vi "ui_DataLog Query Meta.vi"(7 "base tag":string) -> (3 "initial value out":dbl format="%.2f", 4 "OKed?":bool, 8 "meta out":T1)   [LabVIEW 2012]
doc: "This dialog queries meta tag type and initial value."
uses:
  typedefs/et_DataLog Meta Tag Specifier.ctl
  typedefs/t_DataLog Query Meta States.ctl
panel:
  in  "initial value":dbl format="%.4e"
  in  "meta specifier":T1=enum."not a meta"
  in  "cancel":bool
  in  "OK":bool
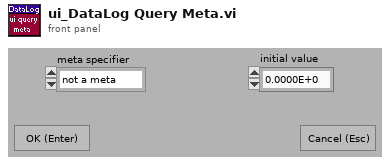
[diagram p1: front panel]
types:
  T1 = typedef "et_DataLog Meta Tag Specifier.ctl" = enum32{"warn_lo", "warn_hi", "A_lo", "A_hi", "B_lo", "B_hi", "C_lo", "C_hi", "D_lo", "D_hi", "E_lo", "E_hi", "F_lo", "F_hi", "G_lo", "G_hi", "H_lo", "H_hi", "I_lo", "I_hi", "J_lo", "J_hi", "K_lo", "K_hi", "L_lo", "L_hi", "M_lo", "M_hi", "N_lo", "N_hi", "min", "max", "not a meta"}
  T2 = typedef "t_DataLog Query Meta States.ctl" = enum16{"empty queue", "initialize", "stop"}
  T3 = typedef "eventvkey.ctl" = enum16{"ASCII", "Enter", "Return", "Shift", "Ctrl", "Alt", "Cmd", "Opt", "Caps", "NumLock", "Clear", "Break", "Up", "Down", "Left", "Right", "Insert", "Delete", "Home", "End", "PageUp", "PageDown", "Escape", "Help", "Pause", "ScrollLock", "F1", "F2", "F3", "F4", "F5", "F6", "F7", "F8", "F9", "F10", "F11", "F12", "F13", "F14", "F15", "F16", "F17", "F18", "F19", "F20", "F21", "F22", "F23", "F24", "Play", "VolumeUp", "VolumeDown", "Mute", "Two Byte Char"}
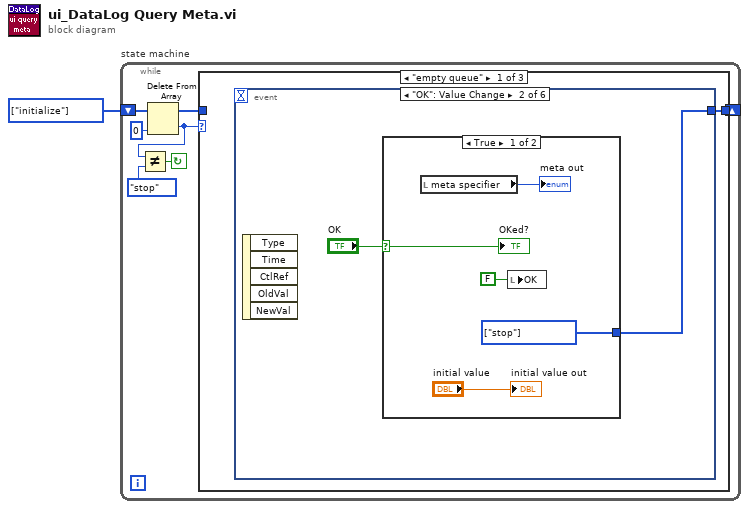
[diagram p0: block diagram]
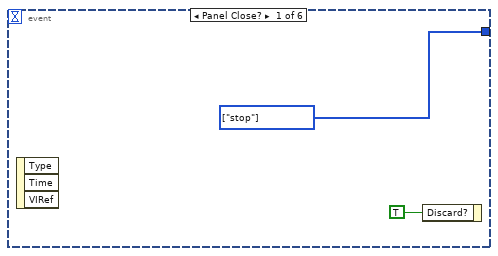
[diagram p2: hidden frame]
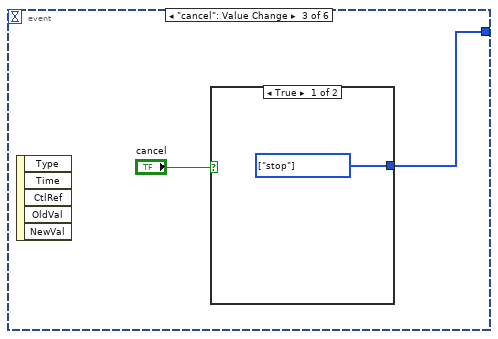
[diagram p4: hidden frame]
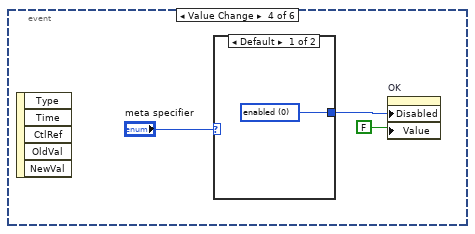
[diagram p6: hidden frame]
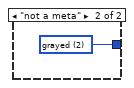
[diagram p7: hidden frame]
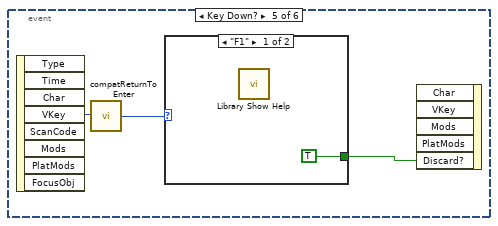
[diagram p8: hidden frame]
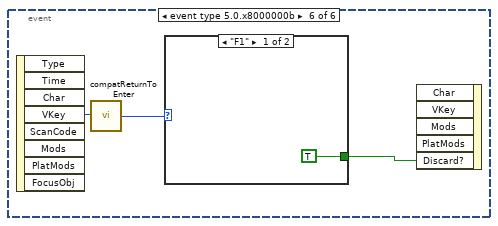
[diagram p10: hidden frame]
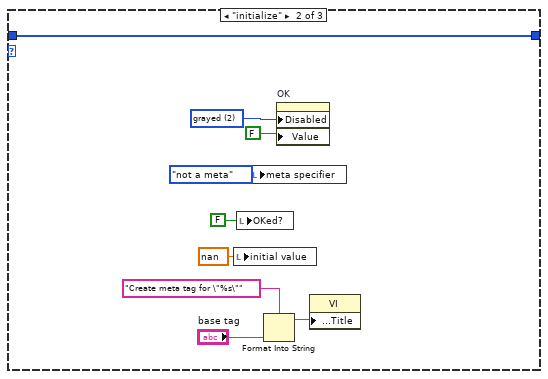
[diagram p12: hidden frame]
diagram:
  w1 = T2[] [enum."initialize"] items=["empty queue", "initialize", "stop"] ("Array Constant")
  n1 = while "state machine" {
    shift-left: w1 -> [w5]
    shift-right: [w8] -> _
    stop <- w7 continue-if-true
    n2 = Delete From Array(array=w5, index=0) -> (deleted portion=w3:T2, array with subset deleted=w4:T2[])  [unwired: 1 in]
    n3 = Not Equal?(x=w3, y=t_DataLog_Query_Meta_States."stop" ("states")) -> (x != y?=w7:bool)
    n4 = case "Case" shown="\"empty queue\"" w3 {
      tunnel: [w9 w43 w44] -> w8
      tunnel: w4 -> [_ w43 w44]
      frame "empty queue" {
        n5 = event shown="[1] \"OK\": Value Change" {
          selector: _ -> [_ _ _ _ _ _]
          dyn-events: _ -> [_ _ _ _ _ _]
          timeout: _ -> [_ _ _ _ _ _]
          tunnel: [w11 w13 w20 _ _ _] -> w9
          event Panel Close? {
            w11 = T2[] [enum."stop"] items=["empty queue", "initialize", "stop"] ("Array Constant")
            n6 = event-data() -> ()  [unwired: 1 in, 3 out]
            n7 = event-data("Discard?"=TRUE) -> ()  [unwired: 1 in, 1 out]
          }
          event "OK": Value Change {
            n8 = event-data() -> ()  [unwired: 1 in, 5 out]
            n9 = case shown="True" "OK" {
              selector: "OK" -> [w17 _]
              tunnel: [w18 _] -> w13
              frame True {
                w18 = T2[] [enum."stop"] items=["empty queue", "initialize", "stop"] ("Array Constant")
                n10 = local read "meta specifier"() -> (→"meta out":T1)
                n11 = local write "OK"(FALSE ("OK")) -> ()
                "OKed?" <- w17
                "initial value out" <- "initial value"
              }
              frame False {
              }
            }
          }
          event "cancel": Value Change {
            n12 = event-data() -> ()  [unwired: 1 in, 5 out]
            n13 = case shown="True" "cancel" {
              tunnel: [w21 _] -> w20
              frame True {
                w21 = T2[] [enum."stop"] items=["empty queue", "initialize", "stop"] ("Array Constant")
              }
              frame False {
              }
            }
          }
          event Value Change {
            n14 = event-data() -> ()  [unwired: 1 in, 5 out]
            n15 = case shown="Default" "meta specifier" {
              tunnel: [w25 w26] -> w22
              frame Default {
                w25 = u8 0 items=["enabled", "disabled", "grayed"] ("disabled state")
              }
              frame "not a meta" {
                w26 = u8 2 items=["enabled", "disabled", "grayed"] ("disabled state")
              }
            }
            n16 = property on="OK" class="Bool (strict)"("Disabled"=w22, "Value"=FALSE ("OK")) -> ()  [unwired: 2 in, 2 out]
          }
          event Key Down? {
            n17 = event-data() -> ("VKey"=w27:T3)  [unwired: 1 in, 7 out]
            n18 = call <vilib>:"compatReturnToEnter.vi"("VKey"=w27) -> ("VKey"=w29:T3)
            n19 = case shown="\"F1\"" w29 {
              tunnel: [TRUE ("Discard?") _] -> w28
              frame "F1" {
                n20 = call "Library Show Help.vi"() -> ()  [unwired: 1 in]
              }
              frame Default {
              }
            }
            n21 = event-data("Discard?"=w28) -> ()  [unwired: 5 in, 1 out]
          }
          event event type 5.0.x8000000b {
            n22 = event-data() -> ("VKey"=w31:T3)  [unwired: 1 in, 7 out]
            n23 = call <vilib>:"compatReturnToEnter.vi"("VKey"=w31) -> ("VKey"=w33:T3)
            n24 = case shown="\"F1\"" w33 {
              tunnel: [TRUE ("Discard?") _] -> w32
              frame "F1" {
              }
              frame Default {
              }
            }
            n25 = event-data("Discard?"=w32) -> ()  [unwired: 5 in, 1 out]
          }
        }
      }
      frame "initialize" {
        w39 = u8 2 items=["enabled", "disabled", "grayed"] ("disabled state")
        n26 = local write "initial value"(nan ("initial value")) -> ()
        n27 = local write "OKed?"(FALSE ("OKed?")) -> ()
        n28 = local write "meta specifier"(et_DataLog_Meta_Tag_Specifier."not a meta" ("meta specifier")) -> ()
        n29 = Format Into String(format string="Create meta tag for \"%s\"", "base tag") -> (resulting string=w35:string)  [unwired: 2 in, 1 out]
        n30 = property on="OK" class="Bool (strict)"("Disabled"=w39, "Value"=FALSE ("OK")) -> ()  [unwired: 2 in, 2 out]
        n31 = property class="VI"("Front Panel Window:Title"=w35) -> ()  [unwired: 2 in, 2 out]
      }
      frame "stop" {
      }
    }
  }
